vi "Node - PXImc Read.vi"(8 "error in (no error)":errorcluster, 11 "Node Data In":T1) -> (0 "error out":errorcluster, 2 "Readers Data Out":u8[](array[numeric]), 3 "Node Data In":T1)   [LabVIEW 2016, in "PXImc Router.lvlib"]
uses:
  PXImc Router.lvlib
  Controls/Node Data.ctl
  <vilib>/NI Veristand/VeriStand Data/Byte Buffer/Byte Buffer.lvclass
  Controls/Node/Node - PXImc Parameters.ctl
  Controls/Node/Node - Writer Data.ctl
  Controls/Node/Node Ch Properties.ctl
  Controls/Data Type.ctl
  Controls/Node/Node - Readers Data.ctl
  Controls/Node/Node - Reader Data.ctl
  <vilib>/pximc/Acquire Read Region (U8).vi
  <resource>/objmgr/pximc.rc
  <vilib>/pximc/nipximc.lvlib
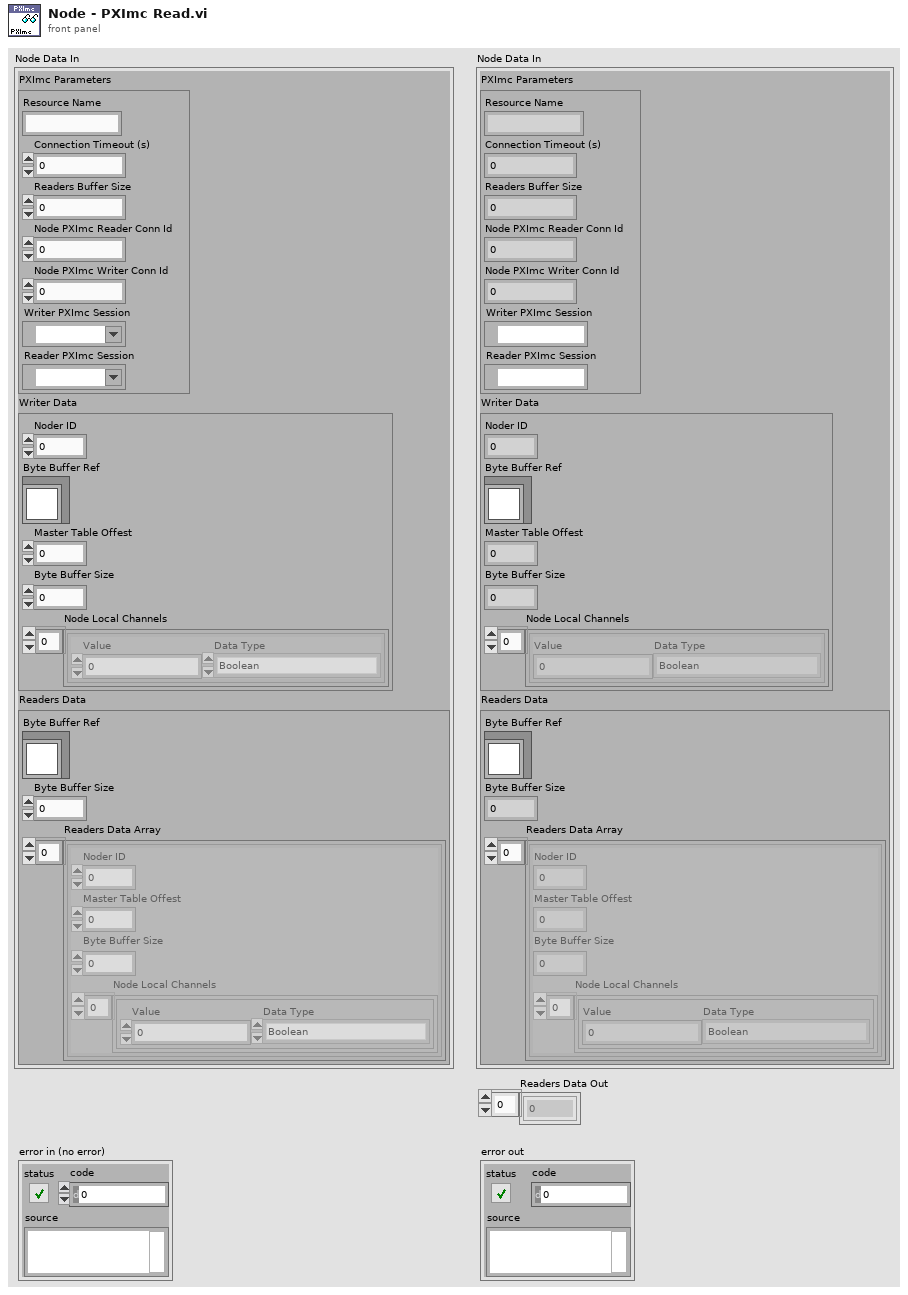
[diagram p1: front panel]
types:
  T1 = typedef "PXImc Router.lvlib/Node Data.ctl" = cluster{"PXImc Parameters":T2, "Writer Data":T3, "Readers Data":T6}
  T2 = typedef "PXImc Router.lvlib/Node - PXImc Parameters.ctl" = cluster{"Resource Name":string, "Connection Timeout (s)":dbl, "Readers Buffer Size":u64, "Node PXImc Reader Conn Id":u16, "Node PXImc Writer Conn Id":u16, "Writer PXImc Session":refnum<k21>, "Reader PXImc Session":refnum<k21>}
  T3 = typedef "PXImc Router.lvlib/Node - Writer Data.ctl" = cluster{"Noder ID":u32, "Byte Buffer Ref":refnum<class "Byte Buffer.lvclass">, "Master Table Offest":u32, "Byte Buffer Size":u32, "Node Local Channels":T4[]}
  T4 = typedef "PXImc Router.lvlib/Node Ch Properties.ctl" = cluster{"Value":dbl, "Data Type":T5}
  T5 = typedef "PXImc Router.lvlib/Data Type.ctl" = enum16{"Boolean", "SGL", "DBL", "I8", "I16", "I32", "I64", "U8", "U16", "U32", "U64"}
  T6 = typedef "PXImc Router.lvlib/Node - Readers Data.ctl" = cluster{"Byte Buffer Ref":refnum<class "Byte Buffer.lvclass">, "Byte Buffer Size":u64, "Readers Data Array":T7[]}
  T7 = typedef "PXImc Router.lvlib/Node - Reader Data.ctl" = cluster{"Noder ID":u32, "Master Table Offest":u32, "Byte Buffer Size":u64, "Node Local Channels":T4[]}
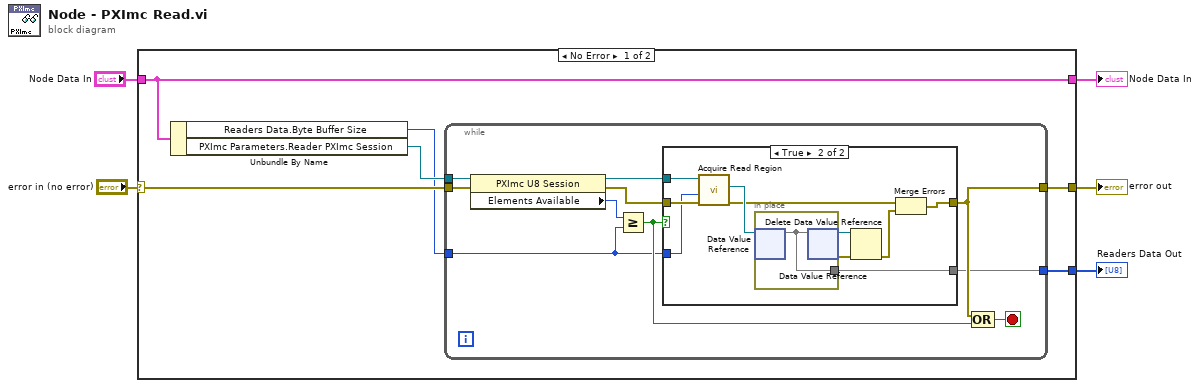
[diagram p0: block diagram]
diagram:
  n1 = case shown="No Error" "error in (no error)" {
    selector: "error in (no error)" -> [w9 w35]
    tunnel: [w8 w35] -> w2
    tunnel: "Node Data In" -> [w11 w34]
    tunnel: [w11 w34] -> w5
    tunnel: [w7 _] -> w1
    frame No Error {
      n2 = Unbundle By Name(w11) -> ("Readers Data.Byte Buffer Size"=w6:u64, "PXImc Parameters.Reader PXImc Session"=w10:refnum<k21>)
      n3 = while {
        tunnel: w9 -> [w19]
        tunnel: [w15] -> w8
        tunnel: [w14] -> w7
        tunnel: w6 -> [w13]
        tunnel: w10 -> [w12]
        stop <- w16 stop-if-true
        n4 = property class="PXImc U8 Session"(reference=w12, error in=w19) -> (reference out=w20:refnum<k21>, error out=w18:errorcluster, "Elements Available"=w21:u64)
        n5 = Greater Or Equal?(x=w21, y=w13) -> (x >= y?=w17:bool)
        n6 = case shown="True" w17 {
          tunnel: w18 -> [w22 w31]
          tunnel: [w22 w25] -> w15
          tunnel: w20 -> [_ w30]
          tunnel: w13 -> [_ w24]
          tunnel: [_ w23] -> w14
          frame False {
          }
          frame True {
            n7 = call-poly <vilib>:"Acquire Read Region.vi"("error in (no error)"=w31, "number of elements"=w24, "session in"=w30) -> ("error out"=w26:errorcluster, "read region reference"=w32:refnum<data-value>)  [unwired: 5 in, 2 out]
            n8 = in-place {
              in-place-border: [w33] -> w23
              n9 = in-place-dvr #1(w32) -> (w33:u8[])  [unwired: 1 out]
              n10 = in-place-dvr #1(w33) -> (w29:refnum<data-value>, w28:errorcluster)
            }
            n11 = Delete Data Value Reference(data value reference=w29, error in=w28) -> (error out=w27:errorcluster)  [unwired: 1 out]
            n12 = Merge Errors(w26, w27) -> (w25:errorcluster)
          }
        }
        n13 = Compound Arithmetic op=OR(w15, w17) -> (w16:bool)
      }
    }
    frame Error {
    }
  }
  "Node Data In" <- w5
  "error out" <- w2
  "Readers Data Out" <- w1
